vi "Clear Device Groups.vi"(8 "error in":errorcluster, 11 "Startup Optimization in":refnum<class "Startup Optimization.lvclass">) -> (0 "error out":errorcluster, 3 "Startup Optimization out":refnum<class "Startup Optimization.lvclass">)   [LabVIEW 2018, in "Startup Optimization Actor.lvlib" / "Startup Optimization.lvclass"]
uses:
  Startup Optimization.lvclass
  Controls/Device Groups.ctl
  <vilib>/ORNL/CSEISMIC DDS/CSEISMIC DDS Base/Data Types/Controls/DeviceID.ctl
  Startup Optimization.lvclass/Startup Optimization.ctl
  <vilib>/ORNL/CSEISMIC DDS/CSEISMIC DDS Base/CSEISMIC DDS.lvclass
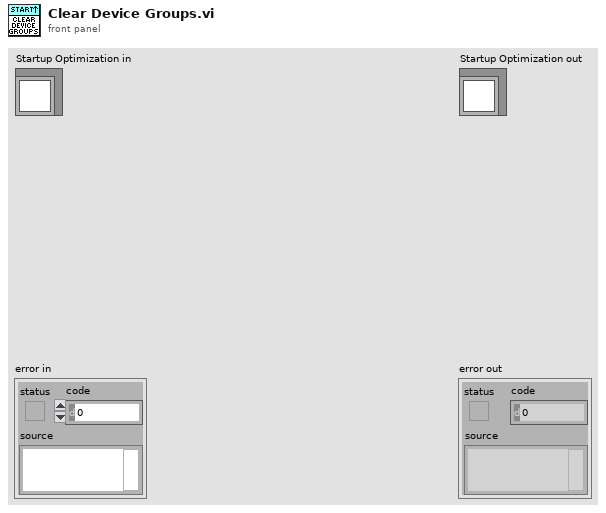
[diagram p1: front panel]
types:
  T1 = typedef "Startup Optimization Actor.lvlib/Startup Optimization.lvclass/Device Groups.ctl" = cluster{"PCC":T2[], "Relays":T2[], "Loads":T2[], "DERs":T2[]}
  T2 = typedef "CSEISMIC DDS.lvlib/CSEISMIC DDS.lvclass/DeviceID.ctl" = string
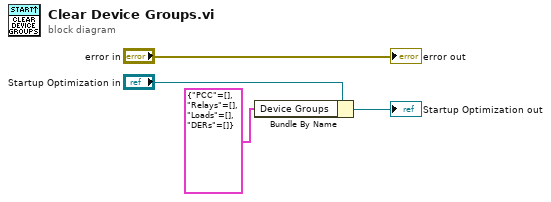
[diagram p0: block diagram]
diagram:
  n1 = Bundle By Name(cluster="Startup Optimization in", "Device Groups"=T1 {"PCC"=[], "Relays"=[], "Loads"=[], "DERs"=[]}) -> (→"Startup Optimization out":refnum<class "Startup Optimization.lvclass">)
  "error out" <- "error in"
